vi "Set Rounding Parameters.vi"(8 "error in (no error)":errorcluster, 9 "Rounding Size":cluster{"Width":i16, "Height":i16}, 10 "Round":bool, 11 "Rectangle in":refnum<class "Rectangle.lvclass">) -> (0 "error out":errorcluster, 3 "Rectangle out":refnum<class "Rectangle.lvclass">)   [LabVIEW 2017, in "LV Image Editor Framework.lvlib" / "Rectangle.lvclass"]
uses:
  Rectangle.lvclass
  Rectangle.lvclass/Rectangle.ctl
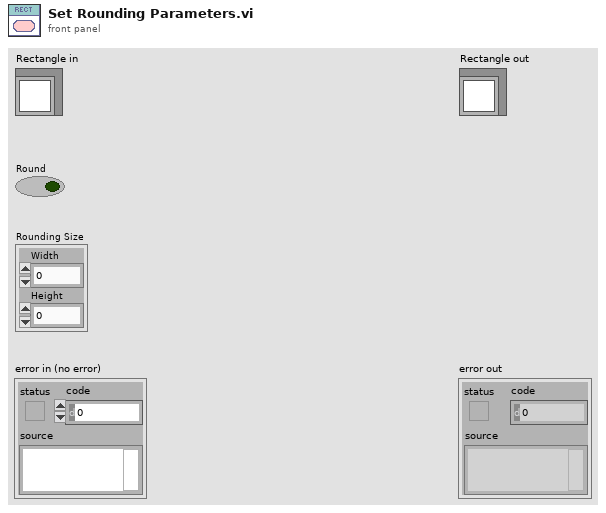
[diagram p1: front panel]
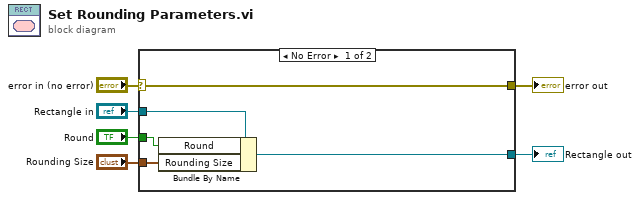
[diagram p0: block diagram]
diagram:
  n1 = case shown="No Error" "error in (no error)" {
    selector: "error in (no error)" -> [w11 w13]
    tunnel: [w11 w13] -> w5
    tunnel: [w9 w12] -> w3
    tunnel: "Rectangle in" -> [w10 w12]
    tunnel: "Round" -> [w8 _]
    tunnel: "Rounding Size" -> [w7 _]
    frame No Error {
      n2 = Bundle By Name(cluster=w10, "Round"=w8, "Rounding Size"=w7) -> (w9:refnum<class "Rectangle.lvclass">)
    }
    frame Error {
    }
  }
  "error out" <- w5
  "Rectangle out" <- w3
